vi "Read Msg Output.vi"(10 "Msg Output":refnum<class "Msg Output.lvclass">) -> ()   [LabVIEW 2020, in "jettl.lvlib" / "Stop jettl Msg.lvlib" / "Stop Msg Output.lvlib"]
uses:
  Stop Msg Output.lvlib
  Msg Output/Msg Output.lvclass
  Stop Msg Output/Stop Msg Output.lvclass
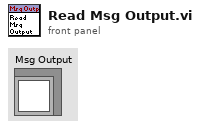
[diagram p1: front panel]
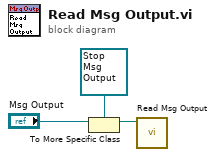
[diagram p0: block diagram]
diagram:
  n1 = To More Specific Class(target class=refnum<class "Stop Msg Output.lvclass"> refnum ("jettl.lvlib:Stop jettl Msg.lvlib:Stop Msg Output.lvlib:Stop Msg Output.lvclass"), reference="Msg Output") -> (specific class reference=w1:refnum<class "Stop Msg Output.lvclass">)  [unwired: 1 in, 1 out]
  n2 = call "Read Msg Output.vi"("Stop Msg Output in"=w1) -> ()  [unwired: 11 in]
